vi "Load Worksheet names.vi"(8 "error in (no error)":errorcluster, 11 "template (empty)":path) -> (0 "error out":errorcluster, 1 "Worksheets names":string[](array[string]), 2 "Worksheets":string[][][](array[string]), 3 "NI_report out":refnum<class "NI_report.lvclass">)   [LabVIEW 2019]
uses:
  <vilib>/Utility/NIReport.llb/NI_report.lvclass
  <vilib>/Utility/NIReport.llb/Report Type.ctl
  <vilib>/addons/_office/excel.llb/Excel Get Data ([str]).vi
  <vilib>/Utility/NIReport.llb/Excel/NI_Excel.lvclass
  <vilib>/addons/_office/NI_ReportGenerationToolkit.lvlib
  <vilib>/Utility/NIReport.llb/NI_ReportGenerationCore.lvlib
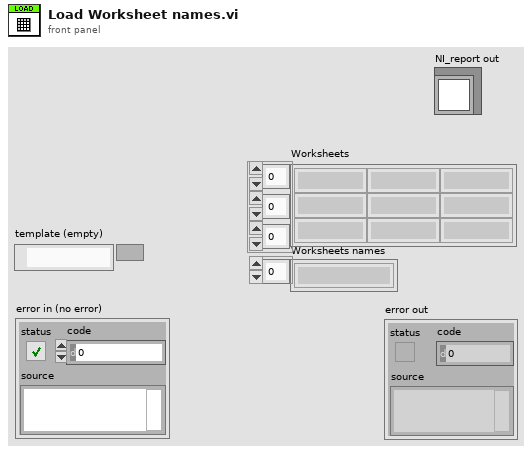
[diagram p1: front panel]
types:
  T1 = typedef "NI_ReportGenerationCore.lvlib/Report Type.ctl" = enum16{"HTML", "Word", "Excel"}
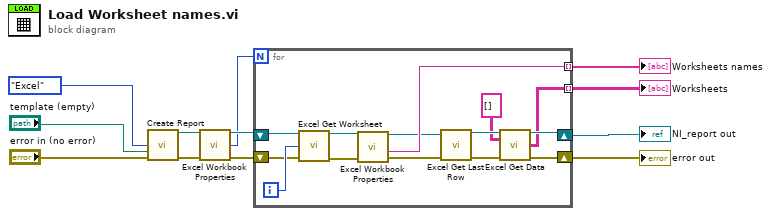
[diagram p0: block diagram]
diagram:
  n1 = call <vilib>:"Create Report.vi"("report type"=Report_Type."Excel", "template (empty)"="template (empty)", "error in (no error)"="error in (no error)") -> ("report out"=w8:refnum<class "NI_report.lvclass">, "error out"=w5:errorcluster)  [unwired: 11 in]
  n2 = call <vilib>:"Excel Workbook Properties.vi"("report in"=w8, "error in (no error)"=w5) -> ("report out"=w7:refnum<class "NI_report.lvclass">, "worksheets count"=w4:i32, "error out"=w6:errorcluster)  [unwired: 10 in, 1 out]
  n3 = for {
    N: w4 -> [_]
    tunnel: [w22] -> w9 mode=indexing
    shift-right: [w15] -> w2
    shift-left: w7 -> [w24]
    shift-right: [w14] -> w1
    shift-left: w6 -> [w21]
    tunnel: [w13] -> w3 mode=indexing
    i -> [w23]
    n4 = call <vilib>:"Excel Get Worksheet.vi"("report in"=w24, "worksheet index (0)"=w23, "error in (no error)"=w21) -> ("report out"=w25:refnum<class "NI_report.lvclass">, "error out"=w26:errorcluster)  [unwired: 11 in]
    n5 = call <vilib>:"Excel Workbook Properties.vi"("report in"=w25, "error in (no error)"=w26) -> ("report out"=w17:refnum<class "NI_report.lvclass">, "current worksheet name"=w22:string, "error out"=w16:errorcluster)  [unwired: 10 in, 1 out]
    n6 = call <vilib>:"Excel Get Last Row.vi"("report in"=w17, "error in (no error)"=w16) -> ("report out"=w19:refnum<class "NI_report.lvclass">, "error out"=w20:errorcluster)  [unwired: 11 in, 1 out]
    n7 = call-poly <vilib>:"Excel Get Data.vi"("report in"=w19, "data type"=string[][] [], "error in (no error)"=w20) -> ("report out"=w15:refnum<class "NI_report.lvclass">, "data"=w13:string[][], "error out"=w14:errorcluster)  [unwired: 10 in]
  }
  "NI_report out" <- w2
  "Worksheets names" <- w9
  "Worksheets" <- w3
  "error out" <- w1
